vi "__Alicat SD_AutoSetFlows.vi"(6 "Cero":bool, 8 "error in (no error)":errorcluster, 10 "ALICATS_SP":T2, 11 "COMMS":T1={"Alicats"="ASRL6::INSTR", "Alic"=FALSE, "eValve"="ASRL6::INSTR", "eval"=FALSE, "Eurotherm"="ASRL6::INSTR", "euro"=FALSE, "Cell GAS"="ASRL6::INSTR", "cgas"=FALSE, "Cell H2S"="ASRL6::INSTR", "ch2s"=FALSE}) -> (0 "error out":errorcluster)   [LabVIEW 2017]
doc: "Use this template to create a dialog box. This template polls the state of the buttons on the front panel and does not use events. Use the Dialog Using Events template (not available in Base package) to create a dialog box with event handling."
uses:
  __s_TablaAlicats.ctl
  __s_SPali4.ctl
  REACTOR_COMUNICACIONES.ctl
  REACTOR_GLOBALES.vi
panel:
  out "Nodos":i32=4
  out "Canal":i32
  out "ID":string[](array[string])
  out "CONECTADO":bool[](array[boolean])
  out "aDispositivos":T3=[["A", "NO", "aM0000013", "Air", "100", "ln/mn", "0.1", "0.11"], ["B", "NO", "aM0000014", "Air", "100", "ln/mn", "0.2", "0.22"], ["C", "NO", "aM0000015", "Air", "100", "ln/mn", "0.3", "0.33"], ["D", "NO", "aM0000016", "Air", "500", "ln/mn", "0.4", "0.44"]] caption="Alicats"
  out "RANGOS":dbl[](array[numeric]) format="%.1g"
  out "SET FLOW":dbl[](array[numeric]) format="%.1f"
  # "Cambio de flujos ALICATS"
  # "Modo automático SP"
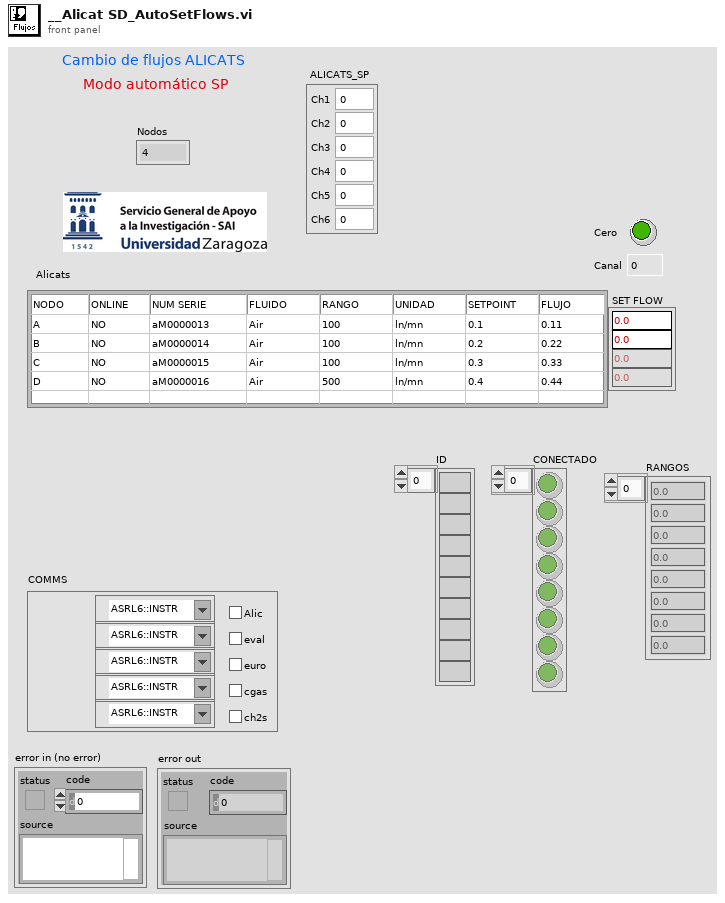
[diagram p1: front panel]
types:
  T1 = typedef "REACTOR_COMUNICACIONES.ctl" = cluster{"Alicats":refnum<visa-resource-name>, "Alic":bool, "eValve":refnum<visa-resource-name>, "eval":bool, "Eurotherm":refnum<visa-resource-name>, "euro":bool, "Cell GAS":refnum<visa-resource-name>, "cgas":bool, "Cell H2S":refnum<visa-resource-name>, "ch2s":bool}
  T2 = typedef "__s_SPali4.ctl" = cluster{"Ch1":dbl, "Ch2":dbl, "Ch3":dbl, "Ch4":dbl, "Ch5":dbl, "Ch6":dbl}
  T3 = typedef "__s_TablaAlicats.ctl" = string[][]
  T4 = cluster{"SETPOINT 2[0]":dbl, "SETPOINT 2[1]":dbl, "SETPOINT 2[2]":dbl, "SETPOINT 2[3]":dbl, "SETPOINT 2[4]":dbl, "SETPOINT 2[5]":dbl}
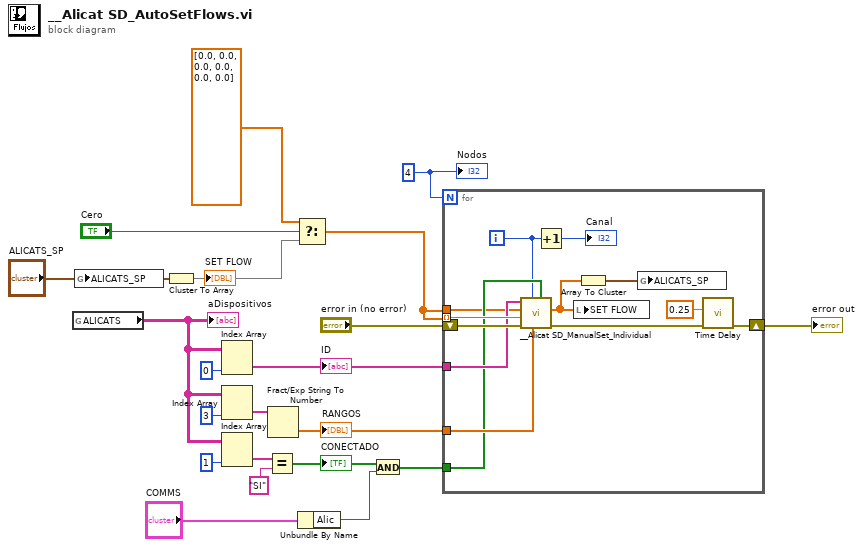
[diagram p0: block diagram]
diagram:
  w1 = 4
  n1 = global read "REACTOR_GLOBALES.vi" "ALICATS"() -> (w8:T3)
  "aDispositivos" <- w8
  n2 = global write "REACTOR_GLOBALES.vi" "ALICATS_SP"("ALICATS_SP") -> ()
  n3 = Cluster To Array(cluster="ALICATS_SP") -> (array=w4:dbl[])
  "SET FLOW" <- w4
  n4 = Index Array(array=w8, index (col)=0 ("disabled index (col)")) -> (element=w13:string[])  [unwired: 1 in]
  "ID" <- w13
  n5 = Index Array(array=w8, index (col)=3 ("disabled index (col)")) -> (element=w20:string[])  [unwired: 1 in]
  n6 = Index Array(array=w8, index (col)=1 ("disabled index (col)")) -> (element=w17:string[])  [unwired: 1 in]
  n7 = Equal?(x=w17, y="SI") -> (x = y?=w11:bool[])
  "CONECTADO" <- w11
  n8 = Fract/Exp String To Number(string=w20) -> (number=w12:dbl[])  [unwired: 3 in, 1 out]
  "RANGOS" <- w12
  n9 = Select(t=dbl[] [0.0, 0.0, 0.0, 0.0, 0.0, 0.0] ("SETPOINTS"), s="Cero", f=w4) -> (s? t:f=w9:dbl[])
  n10 = Unbundle By Name("COMMS") -> ("Alic"=w5:bool)
  n11 = And(x=w11, y=w5) -> (x .and. y?=w6:bool[])
  n12 = for {
    N: w1 -> [_]
    tunnel: w9 -> [w30] mode=indexing
    shift-right: [w31] -> w15
    shift-left: "error in (no error)" -> [w34]
    tunnel: w13 -> [w29]
    tunnel: w12 -> [w28]
    tunnel: w6 -> [w27]
    tunnel: w9 -> [w24]
    i -> [w26]
    n13 = call "__Alicat SD_ManualSet_Individual.vi"("USADO"=w27, "RANGOS"=w28, "Address (0.7)"=w26, "error in"=w34, 9:"SETPOINT"=w30, 10:"SETPOINT"=w24, "ID"=w29) -> ("error out"=w32:errorcluster, "SETPOINT 2"=w23:dbl[])  [unwired: 3 in]
    n14 = Increment(x=w26) -> (x+1=→"Canal":i32)
    n15 = local write "SET FLOW"(w23) -> ()
    n16 = Array To Cluster(array=w23) -> (cluster=w22:T4)
    n17 = global write "REACTOR_GLOBALES.vi" "ALICATS_SP"(w22) -> ()
    n18 = call "Time Delay"("error in (no error)"=w32, "Delay Time (s)"=0.25) -> ("error out"=w31:errorcluster)  [unwired: 9 in]
  }
  "error out" <- w15
  "Nodos" <- w1
